vi "FXP NILIA_PI_LoopFilter.vi"(1 "reset?":bool, 2 "alpha [U16.-2]":fxp<+,16,-2>, 3 "x [I16.2]":fxp<+/-,16,2>) -> (0 "x+y [I32.17]":fxp<+/-,32,17> format="%.21g")   [LabVIEW 2009]
uses:
  <vilib>/rvi/FXPMathLib/FxpMul/XNode/nifxpmath_Multiplier.xnode
  <vilib>/rvi/FXPMathLib/FxpMul/subVIs/nifxpmath_Mul_SimConfig.ctl
  <vilib>/fxp/LVFixedPointQuantizationPolicyTypeDef.ctl
  <vilib>/fxp/LVFixedPointOverflowPolicyTypeDef.ctl
  <vilib>/rvi/FXPMathLib/FxpMul/simVIs/DllFxpMulTemp_sub.vi
  <vilib>/rvi/FXPMathLib/basic elements/FxpIntAccumulator/XNode/nifxpmath_IntAccumulator.xnode
  <vilib>/rvi/FXPMathLib/basic elements/FxpIntAccumulator/subVIs/nifxpmath_IntAccumulator_SimConfig.ctl
  <vilib>/rvi/FXPMathLib/basic elements/FxpIntAccumulator/simVIs/DllFxpIntAccumulator_sub.vi
  <vilib>/rvi/FXPMathLib/FxpAdd/XNode/nifxpmath_Add.xnode
  <vilib>/rvi/FXPMathLib/FxpAdd/subVIs/nifxpmath_Add_SimConfig.ctl
  <vilib>/rvi/FXPMathLib/FxpAdd/simVIs/DllFxpAddTemp_sub.vi
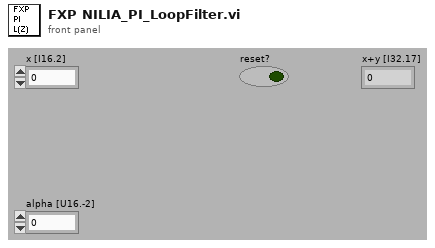
[diagram p1: front panel]
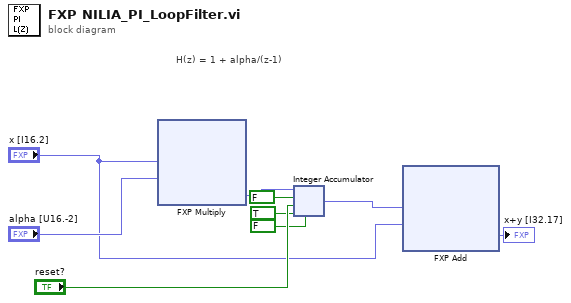
[diagram p0: block diagram]
diagram:
  # "H(z) = 1 + alpha/(z-1)"
  n1 = xnode "FXP Multiply"("x"="x [I16.2]", "y"="alpha [U16.-2]") -> ("x*y"=w4:fxp<+/-,32,0>)
  n2 = xnode "Integer Accumulator"("x"=w4, "load"="reset?", "is sub?"=FALSE ("is sub"), "enable"=TRUE, "carry-in/inverted borrow-in"=FALSE ("cin/nbin")) -> ("s"=w1:fxp<+/-,48,16>)  [unwired: 1 out]
  n3 = xnode "FXP Add"("x"=w1, "y"="x [I16.2]") -> ("x+y"=→"x+y [I32.17]":fxp<+/-,32,17>)
